vi "Add_to_speed_calib_file.vi"(2 "Desired Velocity":dbl format="%.2f", 3 "Max Velocity":dbl format="%.2f", 4 "New Row":dbl[](array[numeric]) format="%.2f", 5 "Tunnel Heated?":bool, 6 "Rig Name":string, 7 "Mode":enum16{"Add Row", "Get Error Value"}(ring)) -> (0 "Tweaked Demand":dbl format="%.4f", 1 "Calib Tweak %":dbl format="%.4f")   [LabVIEW 2010]
uses:
  Anemometry/Anemometry Sub Vis/Controls/In_Range.ctl
  Anemometry/Anemometry Sub Vis/Globals/Constants_global.vi
panel:
  out "Array":dbl[][](array[numeric]) format="%.4f"
  out "Channel Values":string[][](array[string])
  # "Dem Vel       Calib Tweak   Meas Vel"
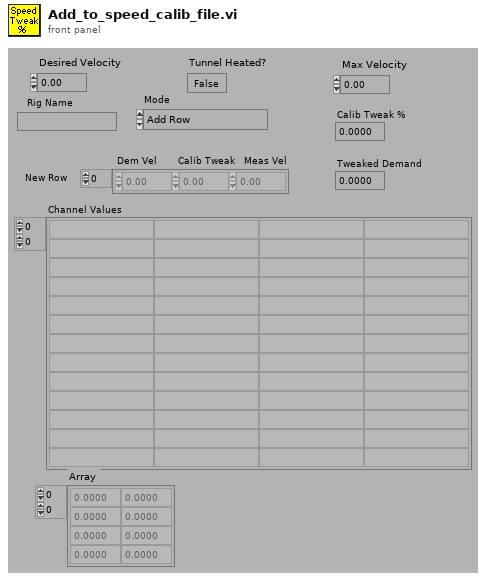
[diagram p1: front panel]
types:
  T1 = typedef "In_Range.ctl" = enum16{"%", "±", "% & ±"}
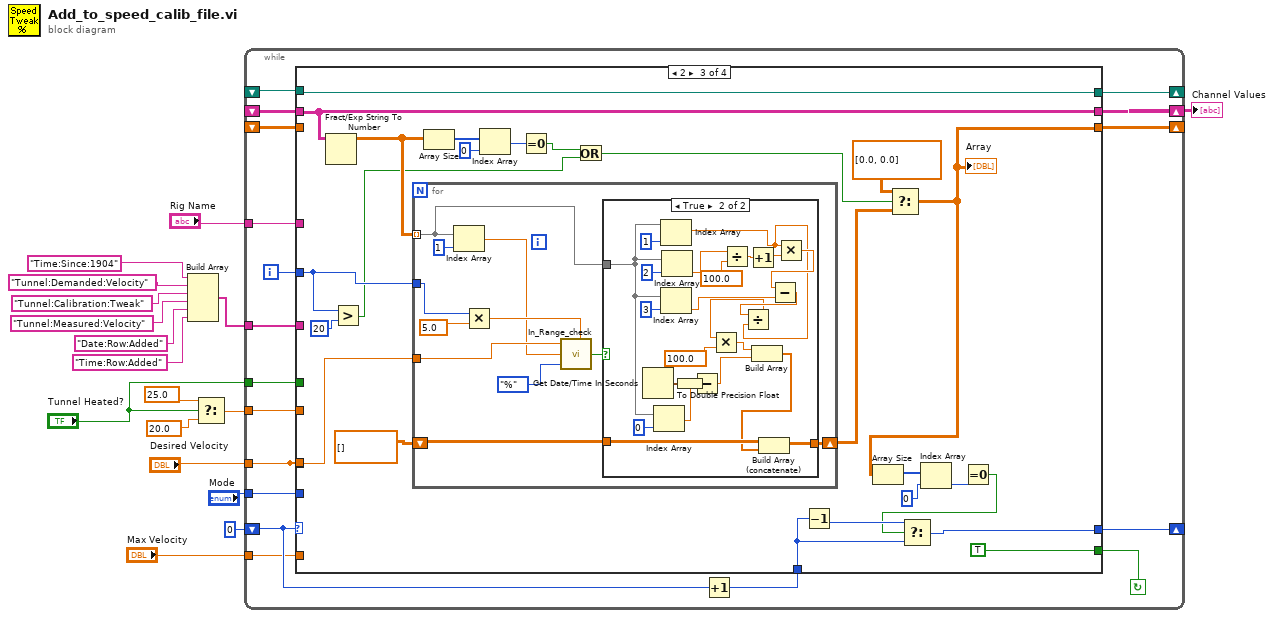
[diagram p0: block diagram]
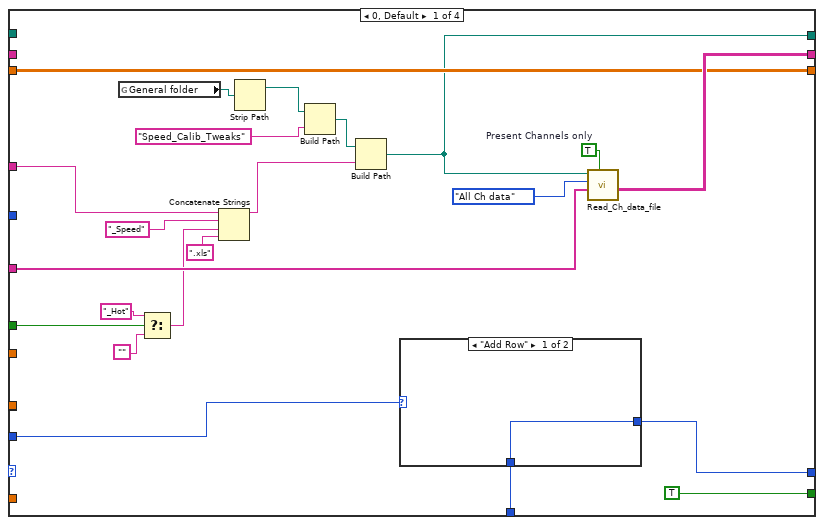
[diagram p2: hidden frame]
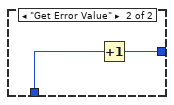
[diagram p3: hidden frame]
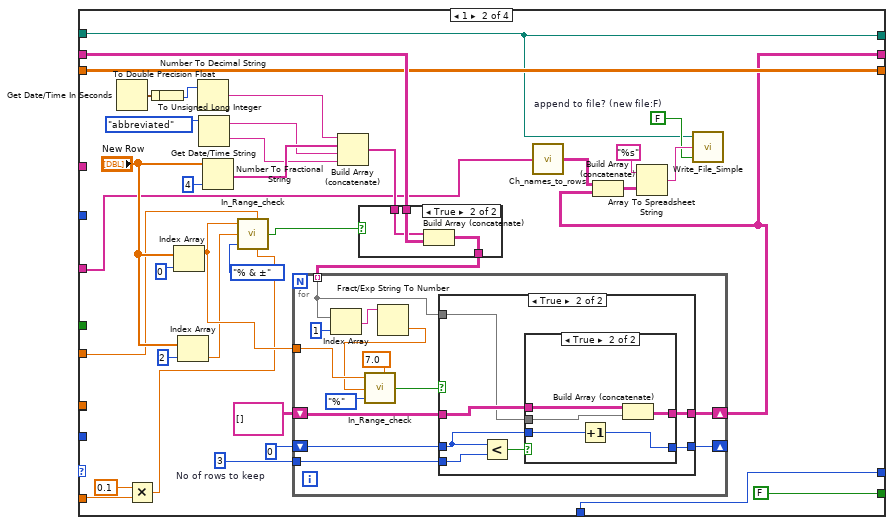
[diagram p4: hidden frame]
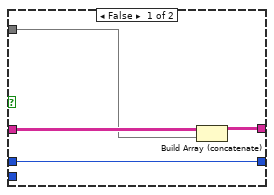
[diagram p6: hidden frame]
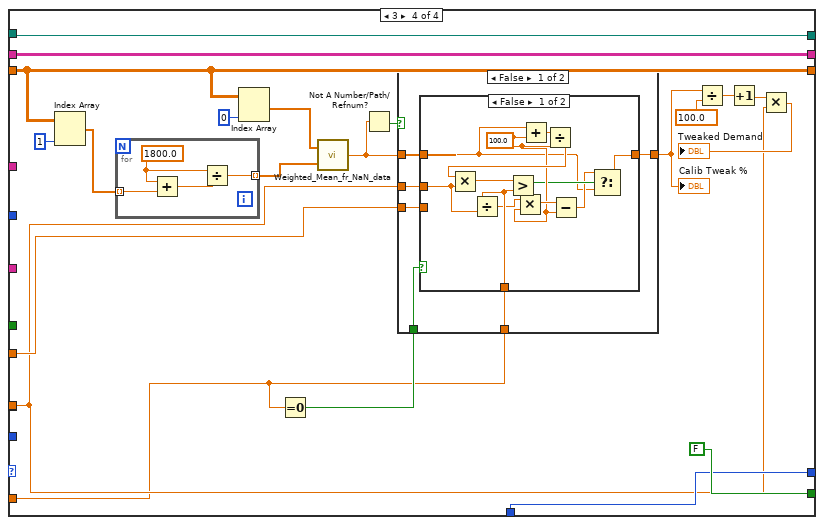
[diagram p9: hidden frame]
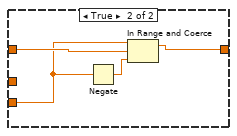
[diagram p10: hidden frame]
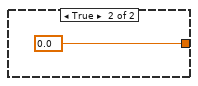
[diagram p11: hidden frame]
diagram:
  n1 = Build Array("Time:Since:1904" ("Substring"), "Tunnel:Demanded:Velocity" ("Substring"), "Tunnel:Calibration:Tweak" ("Substring"), "Tunnel:Measured:Velocity" ("Substring"), "Date:Row:Added" ("Substring"), "Time:Row:Added" ("Substring")) -> (w12:string[])
  n2 = Select(t=25.0 ("Min"), s="Tunnel Heated?", f=20.0 ("Max")) -> (s? t:f=w6:dbl)
  n3 = while {
    tunnel: w6 -> [w19]
    tunnel: "Desired Velocity" -> [w20]
    tunnel: "Tunnel Heated?" -> [w21]
    tunnel: "Rig Name" -> [w22]
    shift-left: _ -> [w23]
    shift-right: [w24] -> _
    tunnel: w12 -> [w30]
    shift-left: _ -> [w27]
    shift-right: [w28] -> w11
    shift-left: _ -> [w26]
    shift-right: [w29] -> _
    tunnel: "Mode" -> [w33]
    shift-left: 0 -> [w34]
    shift-right: [w32] -> _
    tunnel: "Max Velocity" -> [w18]
    i -> [w25]
    stop <- w35 continue-if-true
    n4 = Increment(x=w34) -> (x+1=w31:i32)
    n5 = case shown="2" w34 {
      tunnel: [TRUE FALSE TRUE FALSE] -> w35
      tunnel: w33 -> [w55 _ _ _]
      tunnel: [w54 w87 w153 w207] -> w32
      tunnel: w31 -> [w53 w87 w155 w207]
      tunnel: w30 -> [w52 w66 _ _]
      tunnel: [w37 w67 w152 w212] -> w29
      tunnel: [w51 w65 w151 w211] -> w28
      tunnel: w27 -> [_ w93 w151 w211]
      tunnel: w26 -> [_ w67 w152 w212]
      tunnel: w25 -> [_ _ w140 _]
      tunnel: [w48 w91 w134 w195] -> w24
      tunnel: w23 -> [w48 w91 _ w195]
      tunnel: w22 -> [w47 _ _ _]
      tunnel: w21 -> [w43 _ _ _]
      tunnel: w20 -> [_ _ w144 _]
      tunnel: w20 -> [_ _ _ w194]
      tunnel: w19 -> [_ w61 _ w201]
      tunnel: w18 -> [_ w64 _ w192]
      frame 0, Default {
        w50 = TRUE  # Present Channels only
        n6 = global read "Constants_global.vi" "General folder"() -> (w42:path)
        n7 = Select(t="_Hot", s=w43, f="") -> (s? t:f=w44:string)
        n8 = Concatenate Strings(w47, "_Speed" ("Substring"), w44, ".xls" ("string")) -> (w38:string)
        n9 = Strip Path(path=w42) -> (stripped path=w41:path)  [unwired: 1 out]
        n10 = Build Path(base path=w41, name or relative path="Speed_Calib_Tweaks" ("Input Element")) -> (appended path=w39:path)
        n11 = Build Path(base path=w39, name or relative path=w38) -> (appended path=w37:path)
        n12 = case shown="\"Add Row\"" w55 {
          tunnel: [w58 w59] -> w54
          tunnel: w53 -> [w58 w60]
          frame "Add Row" {
          }
          frame "Get Error Value" {
            n13 = Increment(x=w60) -> (x+1=w59:i32)
          }
        }
        n14 = call "Read_Ch_data_file.vi"("Present Channels only"=w50, "Present Channels"=w52, "Output"=enum16{"All Ch data", "The last few rows"}."All Ch data", "Filename"=w37) -> ("Channel Values"=w51:string[][])  [unwired: 1 in, 4 out]
      }
      frame 1 {
        w68 = FALSE  # append to file? (new file:F)
        w85 = 3  # No of rows to keep
        n15 = Get Date/Time In Seconds() -> (seconds since 1Jan1904=w79:timestamp)
        n16 = Multiply(x=0.1, y=w64) -> (x*y=w62:dbl)
        n17 = To Double Precision Float(number=w79) -> (double precision float=w95:dbl)
        n18 = To Unsigned Long Integer(number=w95) -> (unsigned 32bit integer=w84:u32)
        n19 = Index Array(array="New Row", index=0 ("Index")) -> (element=w76:dbl)
        n20 = Index Array(array="New Row", index=2 ("Index")) -> (element=w75:dbl)
        n21 = Number To Decimal String(number=w84) -> (decimal integer string=w94:string)  [unwired: 1 out]
        n22 = Get Date/Time String(date format (0)=enum16{"short", "long", "abbreviated"}."abbreviated") -> (date string=w82:string, time string=w81:string)  [unwired: 2 out]
        n23 = Number To Fractional String(number="New Row", precision (6)=i16 4) -> (F-format string=w90:string[])  [unwired: 2 out]
        n24 = call "In_Range_check.vi"("±"=w62, "%"=w61, "Mode"=In_Range."% & ±", "Value"=w75, "Setpoint"=w76) -> ("In Range"=w73:bool)  [unwired: 2 out]
        n25 = Build Array (concatenate)(w94, w90, w82, w81) -> (w92:string[])
        n26 = case shown="True" w73 {
          tunnel: w93 -> [w98 w101]
          tunnel: w92 -> [_ w100]
          tunnel: [w98 w99] -> w89
          frame False {
          }
          frame True {
            n27 = Build Array (concatenate)(w100, w101) -> (w99:string[][])
          }
        }
        n28 = for {
          tunnel: w76 -> [w113]
          tunnel: w89 -> [w107] mode=indexing
          shift-right: [w105] -> w65
          shift-left: string[][] [] -> [w106]
          shift-right: [w104] -> _
          shift-left: 0 -> [w103]
          tunnel: w85 -> [w102]
          n29 = Index Array(array=w107, index=1 ("Index")) -> (element=w111:string)
          n30 = Fract/Exp String To Number(string=w111) -> (number=w110:dbl)  [unwired: 4 out]
          n31 = call "In_Range_check.vi"("%"=7.0, "Mode"=In_Range."%", "Value"=w110, "Setpoint"=w113) -> ("In Range"=w108:bool)  [unwired: 1 in, 2 out]
          n32 = case shown="True" w108 {
            tunnel: w107 -> [w117 w123]
            tunnel: w106 -> [w118 w124]
            tunnel: [w116 w122] -> w105
            tunnel: [w115 w120] -> w104
            tunnel: w103 -> [w115 w121]
            tunnel: w102 -> [_ w119]
            frame False {
              n33 = Build Array (concatenate)(w118, w117) -> (w116:string[][])
            }
            frame True {
              n34 = Less?(x=w121, y=w119) -> (x < y?=w125:bool)
              n35 = case shown="True" w125 {
                tunnel: w124 -> [w127 w132]
                tunnel: w123 -> [_ w131]
                tunnel: [w127 w130] -> w122
                tunnel: w121 -> [w126 w129]
                tunnel: [w126 w128] -> w120
                frame False {
                }
                frame True {
                  n36 = Increment(x=w129) -> (x+1=w128:i32)
                  n37 = Build Array (concatenate)(w132, w131) -> (w130:string[][])
                }
              }
            }
          }
        }
        n38 = call "Ch_names_to_rows.vi"("Channel Names"=w66) -> ("3 Row names"=w72:string[][])
        n39 = Build Array (concatenate)(w72, w65) -> (w70:string[][])
        n40 = Array To Spreadsheet String(array=w70, 3:"%s" ("format string")) -> (spreadsheet string=w69:string)  [unwired: 1 out]
        n41 = call "Write_File_Simple.vi"("append to file? (new file:F)"=w68, "character string"=w69, "file path"=w67) -> ()  [unwired: 2 out]
      }
      frame 2 {
        n42 = Fract/Exp String To Number(string=w151) -> (number=w148:dbl[][])  [unwired: 4 out]
        n43 = Greater?(x=w140, y=20) -> (0:w136:bool)
        n44 = for {
          tunnel: w148 -> [w161] mode=indexing
          tunnel: w140 -> [w158]
          tunnel: w144 -> [w166]
          shift-right: [w160] -> w135
          shift-left: dbl[][] [] -> [w162]
          n45 = Index Array(array=w161, index=1 ("Index")) -> (element=w157:dbl)
          n46 = Multiply(x=w158, y=5.0 ("x")) -> (x*y=w164:dbl)
          n47 = call "In_Range_check.vi"("%"=w164, "Mode"=In_Range."%", "Value"=w157, "Setpoint"=w166) -> ("In Range"=w163:bool)  [unwired: 1 in, 2 out]
          n48 = case shown="True" w163 {
            tunnel: w162 -> [w168 w191]
            tunnel: w161 -> [_ w177]
            tunnel: [w168 w190] -> w160
            frame False {
            }
            frame True {
              n49 = Get Date/Time In Seconds() -> (seconds since 1Jan1904=w175:timestamp)
              n50 = Index Array(array=w177, index=0 ("Index")) -> (element=w186:dbl)
              n51 = Index Array(array=w177, index=1 ("Index")) -> (element=w171:dbl)
              n52 = Index Array(array=w177, index=3 ("Index")) -> (element=w173:dbl)
              n53 = Index Array(array=w177, index=2 ("Index")) -> (element=w180:dbl)
              n54 = To Double Precision Float(number=w175) -> (double precision float=w187:dbl)
              n55 = Subtract(x=w187, y=w186) -> (x-y=w185:dbl)
              n56 = Divide(x=w180, y=100.0) -> (x/y=w181:dbl)
              n57 = Increment(x=w181) -> (x+1=w179:dbl)
              n58 = Multiply(x=w171, y=w179) -> (x*y=w174:dbl)
              n59 = Subtract(x=w174, y=w173) -> (x-y=w172:dbl)
              n60 = Divide(x=w172, y=w171) -> (x/y=w169:dbl)
              n61 = Multiply(x=w169, y=100.0) -> (x*y=w170:dbl)
              n62 = Build Array(w170, w185) -> (w184:dbl[])
              n63 = Build Array (concatenate)(w191, w184) -> (w190:dbl[][])
            }
          }
        }
        n64 = Array Size(array=w148) -> (size(s)=w147:i32[])
        n65 = Index Array(array=w147, index=0 ("Index")) -> (element=w145:i32)
        n66 = Equal To 0?(x=w145) -> (x = 0?=w138:bool)
        n67 = Or(x=w138, y=w136) -> (x .or. y?=w137:bool)
        n68 = Decrement(x=w155) -> (x-1=w154:i32)
        n69 = Select(t=dbl[][] [[0.0, 0.0]], s=w137, f=w135) -> (s? t:f=w134:dbl[][])
        "Array" <- w134
        n70 = Array Size(array=w134) -> (size(s)=w143:i32[])
        n71 = Index Array(array=w143, index=0 ("Index")) -> (element=w142:i32)
        n72 = Equal To 0?(x=w142) -> (x = 0?=w133:bool)
        n73 = Select(t=w154, s=w133, f=w155) -> (s? t:f=w153:i32)
      }
      frame 3 {
        n74 = Index Array(array=w195, index (col)=1 ("Index")) -> (element=w203:dbl[])  [unwired: 1 in]
        n75 = for {
          tunnel: w203 -> [w216] mode=indexing
          tunnel: [w213] -> w202 mode=indexing
          w214 = 1800.0
          n76 = Add(x=w214, y=w216) -> (x+y=w215:dbl)
          n77 = Divide(x=w214, y=w215) -> (x/y=w213:dbl)
        }
        n78 = Index Array(array=w195, index (col)=0 ("Index")) -> (element=w204:dbl[])  [unwired: 1 in]
        n79 = Equal To 0?(x=w192) -> (x = 0?=w193:bool)
        n80 = call "Weighted_Mean_fr_NaN_data.vi"("Weighting"=w202, "Data"=w204) -> ("Mean value"=w208:dbl)
        n81 = Not A Number/Path/Refnum?(number/path/refnum=w208) -> (NaN/Path/Refnum?=w209:bool)
        n82 = case shown="False" w209 {
          tunnel: w208 -> [w220 _]
          tunnel: [w219 0.0 ("Clamped output")] -> w200
          tunnel: w201 -> [w217 _]
          tunnel: w194 -> [w222 _]
          tunnel: w192 -> [w221 _]
          tunnel: w193 -> [w218 _]
          frame False {
            n83 = case shown="False" w218 {
              tunnel: w222 -> [w231 _]
              tunnel: w221 -> [w230 _]
              tunnel: w220 -> [w224 w238]
              tunnel: [w223 w235] -> w219
              tunnel: w217 -> [_ w237]
              frame False {
                w227 = 100.0 ("y")
                n84 = Divide(x=w230, y=w231) -> (x/y=w229:dbl)
                n85 = Multiply(x=w229, y=w227) -> (x*y=w228:dbl)
                n86 = Add(x=w224, y=w227) -> (x+y=w234:dbl)
                n87 = Divide(x=w234, y=w227) -> (x/y=w233:dbl)
                n88 = Multiply(x=w233, y=w231) -> (x*y=w232:dbl)
                n89 = Greater?(x=w232, y=w230) -> (0:w226:bool)
                n90 = Subtract(x=w228, y=w227) -> (x-y=w225:dbl)
                n91 = Select(t=w225, s=w226, f=w224) -> (s? t:f=w223:dbl)
              }
              frame True {
                n92 = Negate(x=w237) -> (-x=w236:dbl)
                n93 = In Range and Coerce(upper limit=w237, x=w238, lower limit=w236) -> (coerced(x)=w235:dbl)  [unwired: 1 out]
              }
            }
          }
          frame True {
          }
        }
        "Calib Tweak %" <- w200
        n94 = Divide(x=w200, y=100.0) -> (x/y=w198:dbl)
        n95 = Increment(x=w198) -> (x+1=w197:dbl)
        n96 = Multiply(x=w197, y=w194) -> (x*y=→"Tweaked Demand":dbl)
      }
    }
  }
  "Channel Values" <- w11
